vi "Get Value of LabVIEW Base Type.vi"(1 "LabVIEW Base Type":refnum<vi>, 3 "error in (no error)":errorcluster) -> (7 "JSON Tree Out":variant, 10 "error out":errorcluster)   [LabVIEW 2010, in "i3-json.lvlib"]
doc: "This VI takes a JSON Node (all types besides JSON Object) and assigns the value to the LabVIEW Base Type of compatible reference.\n\nIf the LabVIEW base type is an array of boolean, numeric, or string this function will attempt to check if a JSON Array type will map"
uses:
  i3-json.lvlib
  JSON Types/JSON Type.ctl
  JSON Types/JSON Compatible Type.ctl
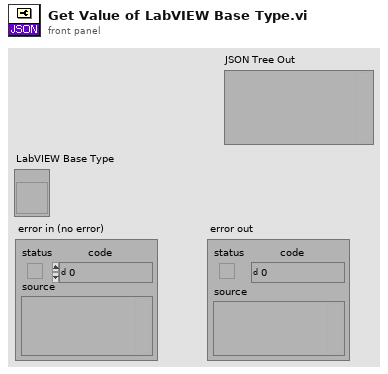
[diagram p1: front panel]
types:
  T1 = typedef "i3-json.lvlib/JSON Type.ctl" = enum8{"JSON Compatible", "JSON Array", "JSON Object", "JSON Null", "Double", "String", "Boolean", "Unknown"}
  T2 = typedef "i3-json.lvlib/JSON Compatible Type.ctl" = enum16{"1D Double Array", "1D String Array", "1D Boolean Array", "Unknown"}
  T3 = typedef "Type Enum.ctl" = enum8{"Void", "I8", "I16", "I32", "I64", "U8", "U16", "U32", "U64", "Single Float", "Double Float", "Extended Float", "Single Complex", "Double Complex", "Extended Complex", "Enum I8 NEVER", "Enum I16 NEVER", "Enum I32 NEVER", "Enum I64 NEVER", "Enum U8", "Enum U16", "Enum U32", "Enum U64", "Single Float With Unit", "Double Float With Unit", "Extended Float With Unit", "Single Complex With Unit", "Double Complex With Unit", "Extended Complex With Unit", "boolU16", "Boolean", "String", "Handle", "Path", "Picture", "C String", "Pascal String", "Tag", "SubString", "Array", "SubArray", "Cluster", "Numeric Cluster", "Variant", "LV Variant", "Measure Data (waveform)", "Refnum", "ExtData", "function", "Typedef", "Poly VI", "bad wire", "LabVIEW Class Instance"}
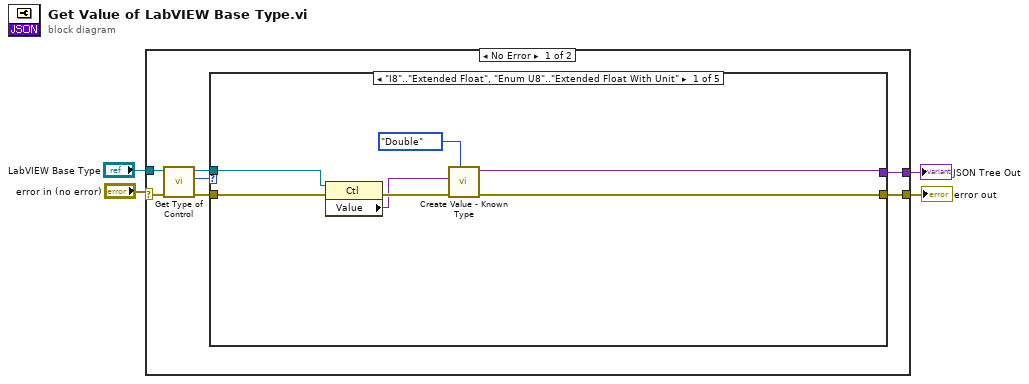
[diagram p0: block diagram]
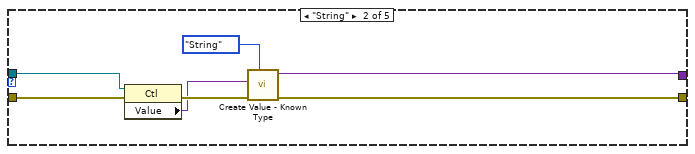
[diagram p2: hidden frame]
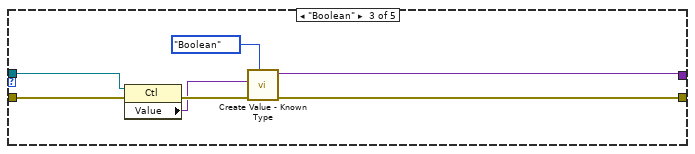
[diagram p3: hidden frame]
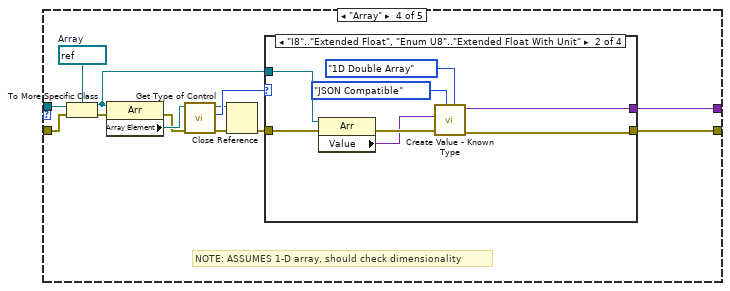
[diagram p4: hidden frame]
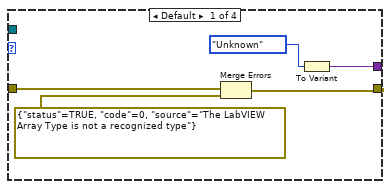
[diagram p5: hidden frame]
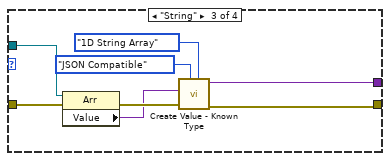
[diagram p6: hidden frame]
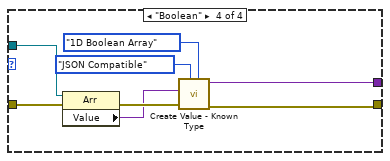
[diagram p7: hidden frame]
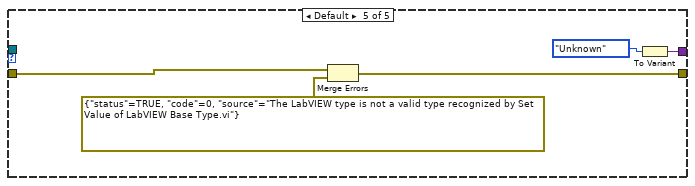
[diagram p8: hidden frame]
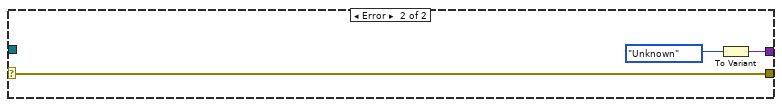
[diagram p9: hidden frame]
diagram:
  n1 = case shown="No Error" "error in (no error)" {
    selector: "error in (no error)" -> [w11 w82]
    tunnel: "LabVIEW Base Type" -> [w10 _]
    tunnel: [w6 w82] -> w2
    tunnel: [w5 w81] -> w1
    frame No Error {
      n2 = call <vilib>:"Get Type of Control.vi"("error in (no error)"=w11, "Control Ref In"=w10) -> ("error out"=w7:errorcluster, "Type Enum"=w9:T3, "Control Ref Out"=w8:refnum<vi>)  [unwired: 7 in]
      n3 = case shown="\"I8\"..\"Extended Float\", \"Enum U8\"..\"Extended Float With Unit\"" w9 {
        tunnel: w8 -> [w17 w24 w31 w44 _]
        tunnel: w7 -> [w18 w25 w32 w45 w79]
        tunnel: [w15 w22 w29 w33 w78] -> w6
        tunnel: [w13 w20 w27 w34 w76] -> w5
        frame "I8".."Extended Float", "Enum U8".."Extended Float With Unit" {
          n4 = property class="Ctl"(reference=w17, error in=w18) -> (error out=w16:errorcluster, "Value"=w14:variant)  [unwired: 1 out]
          n5 = call "Create Value - Known Type.vi"("JSON Type"=JSON_Type."Double", "error in (no error)"=w16, "Value"=w14) -> ("error out"=w15:errorcluster, "JSON Tree"=w13:variant)  [unwired: 7 in]
        }
        frame "String" {
          n6 = property class="Ctl"(reference=w24, error in=w25) -> (error out=w23:errorcluster, "Value"=w21:variant)  [unwired: 1 out]
          n7 = call "Create Value - Known Type.vi"("JSON Type"=JSON_Type."String", "error in (no error)"=w23, "Value"=w21) -> ("error out"=w22:errorcluster, "JSON Tree"=w20:variant)  [unwired: 7 in]
        }
        frame "Boolean" {
          n8 = property class="Ctl"(reference=w31, error in=w32) -> (error out=w30:errorcluster, "Value"=w28:variant)  [unwired: 1 out]
          n9 = call "Create Value - Known Type.vi"("JSON Type"=JSON_Type."Boolean", "error in (no error)"=w30, "Value"=w28) -> ("error out"=w29:errorcluster, "JSON Tree"=w27:variant)  [unwired: 7 in]
        }
        frame "Array" {
          w39 = refnum<vi> refnum  # Array
          # "NOTE: ASSUMES 1-D array, should check dimensionality"
          n10 = To More Specific Class(target class=w39, reference=w44, error in=w45) -> (specific class reference=w35:refnum<vi>, error out=w43:errorcluster)
          n11 = property class="Arr"(reference=w35, error in=w43) -> (error out=w41:errorcluster, "Array Element"=w42:refnum<vi>)  [unwired: 1 out]
          n12 = call <vilib>:"Get Type of Control.vi"("error in (no error)"=w41, "Control Ref In"=w42) -> ("error out"=w38:errorcluster, "Type Enum"=w40:T3, "Control Ref Out"=w36:refnum<vi>)  [unwired: 7 in]
          n13 = Close Reference(reference=w36, error in (no error)=w38) -> (error out=w37:errorcluster)
          n14 = case shown="\"I8\"..\"Extended Float\", \"Enum U8\"..\"Extended Float With Unit\"" w40 {
            tunnel: w37 -> [w50 w57 w65 w73]
            tunnel: [w48 w55 w63 w71] -> w33
            tunnel: w35 -> [_ w58 w66 w74]
            tunnel: [w47 w53 w61 w69] -> w34
            frame Default {
              n15 = Merge Errors(w50, errorcluster {"status"=TRUE, "code"=0, "source"="The LabVIEW Array Type is not a recognized type"} ("error in")) -> (w48:errorcluster)
              n16 = To Variant(anything=JSON_Type."Unknown" ("JSON Type")) -> (Variant=w47:variant)
            }
            frame "I8".."Extended Float", "Enum U8".."Extended Float With Unit" {
              n17 = property class="Arr"(reference=w58, error in=w57) -> (error out=w56:errorcluster, "Value"=w54:variant)  [unwired: 1 out]
              n18 = call "Create Value - Known Type.vi"("JSON Compatible Type"=JSON_Compatible_Type."1D Double Array", "JSON Type"=JSON_Type."JSON Compatible", "error in (no error)"=w56, "Value"=w54) -> ("error out"=w55:errorcluster, "JSON Tree"=w53:variant)  [unwired: 6 in]
            }
            frame "String" {
              n19 = property class="Arr"(reference=w66, error in=w65) -> (error out=w64:errorcluster, "Value"=w62:variant)  [unwired: 1 out]
              n20 = call "Create Value - Known Type.vi"("JSON Compatible Type"=JSON_Compatible_Type."1D String Array", "JSON Type"=JSON_Type."JSON Compatible", "error in (no error)"=w64, "Value"=w62) -> ("error out"=w63:errorcluster, "JSON Tree"=w61:variant)  [unwired: 6 in]
            }
            frame "Boolean" {
              n21 = property class="Arr"(reference=w74, error in=w73) -> (error out=w72:errorcluster, "Value"=w70:variant)  [unwired: 1 out]
              n22 = call "Create Value - Known Type.vi"("JSON Compatible Type"=JSON_Compatible_Type."1D Boolean Array", "JSON Type"=JSON_Type."JSON Compatible", "error in (no error)"=w72, "Value"=w70) -> ("error out"=w71:errorcluster, "JSON Tree"=w69:variant)  [unwired: 6 in]
            }
          }
        }
        frame Default {
          n23 = Merge Errors(w79, errorcluster {"status"=TRUE, "code"=0, "source"="The LabVIEW type is not a valid type recognized by Set Value of LabVIEW Base Type.vi"} ("error in")) -> (w78:errorcluster)
          n24 = To Variant(anything=JSON_Type."Unknown" ("JSON Type")) -> (Variant=w76:variant)
        }
      }
    }
    frame Error {
      n25 = To Variant(anything=JSON_Type."Unknown" ("JSON Type")) -> (Variant=w81:variant)
    }
  }
  "JSON Tree Out" <- w1
  "error out" <- w2
